vi "Exercise 5.1 Webservice.vi"() -> ()   [LabVIEW 2014]
uses:
  <vilib>/Q-Wave Systems/QwaveSys RPi Training Package (Demo)/Addons/WiringPi/WiringPi GPIO TypeDef.ctl
  <vilib>/Q-Wave Systems/QwaveSys RPi Training Package (Demo)/Addons/WiringPi/WiringPi Pin Mode.ctl
  <vilib>/Q-Wave Systems/QwaveSys RPi Training Package (Demo)/Addons/QwaveSys RPi Training Library.lvlib
panel:
  out "Active":bool
  in  "LED2":T1=5 items=["Pin1_3.3V"=51, "Pin2_5V"=52, "Pin3_GPIO8_I2C1_SDA"=8, "Pin4_5V"=53, "Pin5_GPIO9_I2C1_SCL"=9, "Pin6_Gnd"=54, "Pin7_GPIO7_GPCLK0"=7, "Pin8_GPIO15_TXD_UART"=15, "Pin9_Gnd"=55, "Pin10_GPIO16_RXD_UART"=16, "Pin11_GPIO0"=0, "Pin12_GPIO1_PCMCLK_PWM0"=1, "Pin13_GPIO2"=2, "Pin14_Gnd"=56, "Pin15_GPIO3"=3, "Pin16_GPIO4"=4, "Pin17_3V"=57, "Pin18_GPIO5"=5, "Pin19_GPIO12_MOSI(SPI)"=12, "Pin20_Gnd"=58, "Pin21_GPIO13_MISO(SPI)"=13, "Pin22_GPIO6"=6, "Pin23_GPIO14_CLK(SPI)"=14, "Pin24_GPIO10_CE0_SPI"=10, "Pin25_Gnd"=59, "Pin26_GPIO11_CE1_SPI"=11, "Pin27_SDA0_I2C_EEPROM"=60, "Pin28_SCL0_I2C_EEPROM"=61, "Pin_29_GPIO21_GPCLK1"=21, "Pin30_Gnd"=62, "Pin31_GPIO22_GPCLK2"=22, "Pin32_GPIO26_PWM0"=26, "Pin33_GPIO23_PWM1"=23, "Pin34_Gnd"=63, "Pin35_GPIO24_PCMFS_PWM1"=24, "Pin36_GPIO27"=27, "Pin37_GPIO25"=25, "Pin38_GPIO28_PCM_DIN"=28, "Pin39_Gnd"=64, "Pin40_GPIO29_PCM_DOUT"=29]
  in  "LED1":T1=1 items=["Pin1_3.3V"=51, "Pin2_5V"=52, "Pin3_GPIO8_I2C1_SDA"=8, "Pin4_5V"=53, "Pin5_GPIO9_I2C1_SCL"=9, "Pin6_Gnd"=54, "Pin7_GPIO7_GPCLK0"=7, "Pin8_GPIO15_TXD_UART"=15, "Pin9_Gnd"=55, "Pin10_GPIO16_RXD_UART"=16, "Pin11_GPIO0"=0, "Pin12_GPIO1_PCMCLK_PWM0"=1, "Pin13_GPIO2"=2, "Pin14_Gnd"=56, "Pin15_GPIO3"=3, "Pin16_GPIO4"=4, "Pin17_3V"=57, "Pin18_GPIO5"=5, "Pin19_GPIO12_MOSI(SPI)"=12, "Pin20_Gnd"=58, "Pin21_GPIO13_MISO(SPI)"=13, "Pin22_GPIO6"=6, "Pin23_GPIO14_CLK(SPI)"=14, "Pin24_GPIO10_CE0_SPI"=10, "Pin25_Gnd"=59, "Pin26_GPIO11_CE1_SPI"=11, "Pin27_SDA0_I2C_EEPROM"=60, "Pin28_SCL0_I2C_EEPROM"=61, "Pin_29_GPIO21_GPCLK1"=21, "Pin30_Gnd"=62, "Pin31_GPIO22_GPCLK2"=22, "Pin32_GPIO26_PWM0"=26, "Pin33_GPIO23_PWM1"=23, "Pin34_Gnd"=63, "Pin35_GPIO24_PCMFS_PWM1"=24, "Pin36_GPIO27"=27, "Pin37_GPIO25"=25, "Pin38_GPIO28_PCM_DIN"=28, "Pin39_Gnd"=64, "Pin40_GPIO29_PCM_DOUT"=29]
  out "error out":errorcluster
  in  "error in (no error)":errorcluster
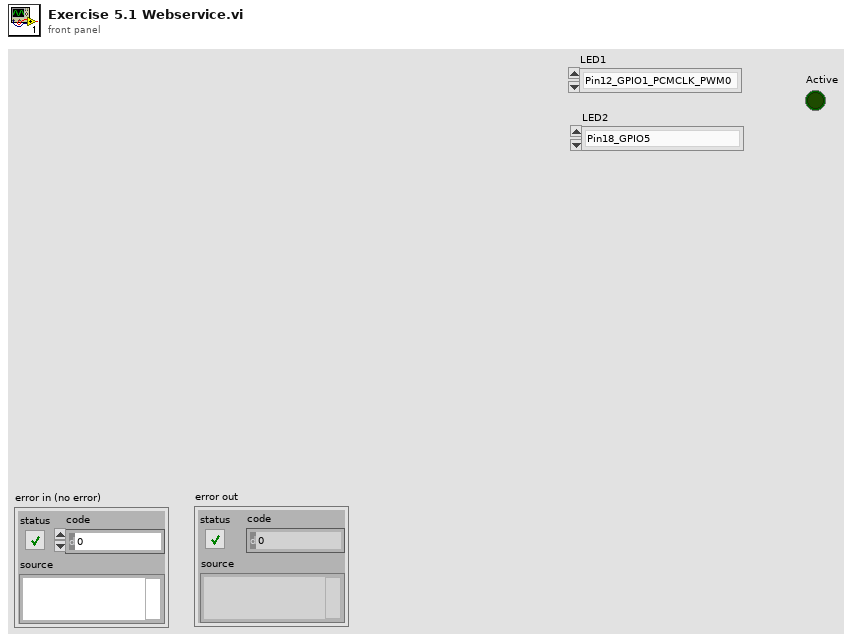
[diagram p1: front panel]
types:
  T1 = typedef "QwaveSys RPi Training Library.lvlib/WiringPi GPIO TypeDef.ctl" = u8
  T2 = typedef "QwaveSys RPi Training Library.lvlib/WiringPi Pin Mode.ctl" = enum8{"INPUT", "OUTPUT", "PWM_OUTPUT", "GPIO_CLOCK", "SOFT_PWM_OUTPUT", "SOFT_TONE_OUTPUT", "PWM_TONE_OUTPUT"}
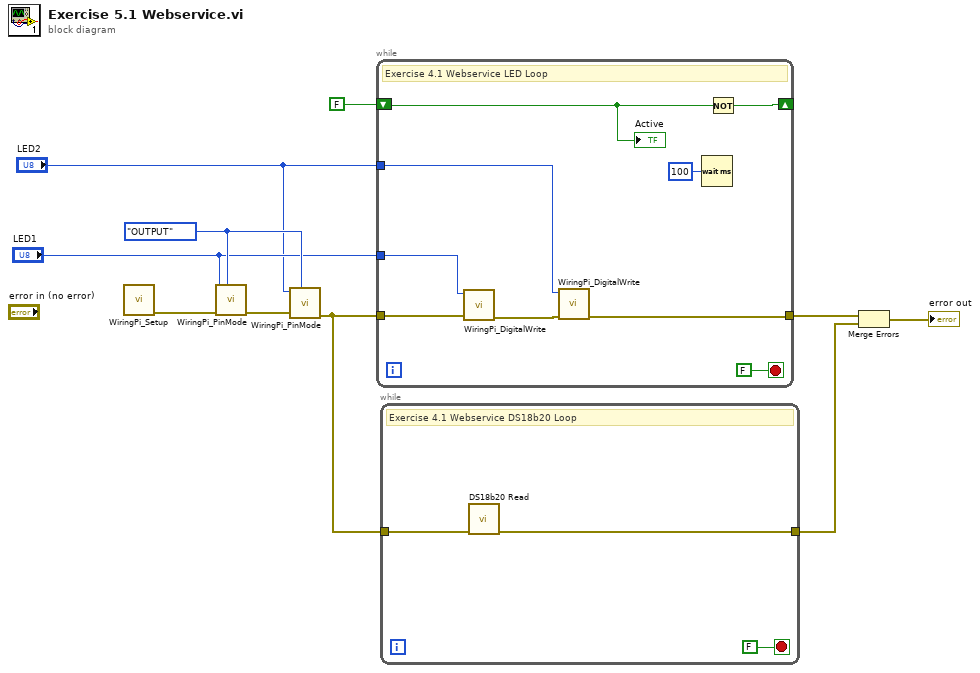
[diagram p0: block diagram]
diagram:
  w8 = WiringPi_Pin_Mode."OUTPUT" ("Pin Mode")
  n1 = call <vilib>:"WiringPi_Setup.vi"() -> ("error out"=w10:errorcluster)  [unwired: 11 in]
  n2 = call <vilib>:"WiringPi_PinMode.vi"("Pin Mode"=w8, "error in (no error)"=w10, "WiringPi GPIO"="LED1") -> ("error out"=w9:errorcluster)  [unwired: 8 in]
  n3 = call <vilib>:"WiringPi_PinMode.vi"("Pin Mode"=w8, "error in (no error)"=w9, "WiringPi GPIO"="LED2") -> ("error out"=w5:errorcluster)  [unwired: 8 in]
  n4 = while {
    tunnel: w5 -> [w18]
    tunnel: "LED1" -> [w17]
    tunnel: "LED2" -> [w16]
    tunnel: [w15] -> w4
    shift-right: [w12] -> _
    shift-left: FALSE -> [w11]
    stop <- FALSE stop-if-true
    # "Exercise 4.1 Webservice LED Loop"
    n5 = call <vilib>:"WiringPi_DigitalWrite.vi"("error in (no error)"=w18, "WiringPi GPIO"=w17) -> ("error out"=w19:errorcluster)  [unwired: 9 in]
    n6 = call <vilib>:"WiringPi_DigitalWrite.vi"("error in (no error)"=w19, "WiringPi GPIO"=w16) -> ("error out"=w15:errorcluster)  [unwired: 9 in]
    n7 = Wait (ms)(milliseconds to wait=u32 100) -> ()  [unwired: 1 out]
    n8 = Not(x=w11) -> (.not. x?=w12:bool)
    "Active" <- w11
  }
  n9 = while {
    tunnel: w5 -> [w22]
    tunnel: [w21] -> w3
    stop <- FALSE stop-if-true
    # "Exercise 4.1 Webservice DS18b20 Loop"
    n10 = call <vilib>:"DS18b20 Read.vi"("error in (no error)"=w22) -> ("error out"=w21:errorcluster)  [unwired: 7 in, 3 out]
  }
  n11 = Merge Errors(w4, w3) -> (→"error out":errorcluster)
